vi "test_BuildAdvancedAssets.vi"() -> (3 "Pass?":bool)   [LabVIEW 2019, in "Tests.SolutionBuilder.lvlib"]
uses:
  Tests.SolutionBuilder.lvlib
panel:
  out "test results":u32 format="%03b"
  out "error out":errorcluster
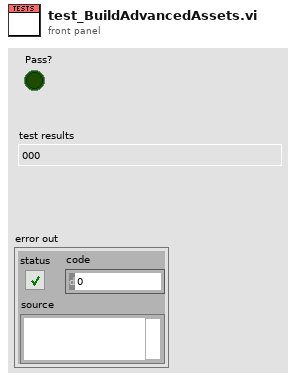
[diagram p1: front panel]
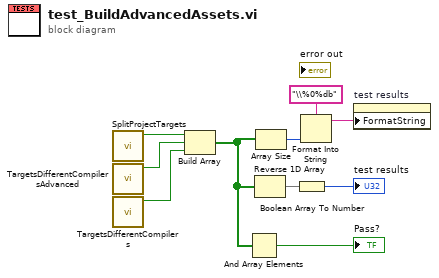
[diagram p0: block diagram]
diagram:
  n1 = call "SplitProjectTargets.vi"() -> ("Pass?"=w6:bool)  [unwired: 11 in]
  n2 = call "TargetsDifferentCompilersAdvanced.vi"() -> ("Pass?"=w1:bool)  [unwired: 10 in, 1 out]
  n3 = call "TargetsDifferentCompilers.vi"() -> ("Pass?"=w5:bool)  [unwired: 11 in]
  n4 = Build Array(w6, w1, w5) -> (w10:bool[])
  n5 = And Array Elements(Boolean array=w10) -> (logical AND=→"Pass?":bool)
  n6 = Reverse 1D Array(array=w10) -> (reversed array=w7:bool[])
  n7 = Array Size(array=w10) -> (size(s)=w8:i32)
  n8 = Boolean Array To Number(Boolean array=w7) -> (number=→"test results":u32)
  n9 = Format Into String(format string="\\%0%db", w8) -> (resulting string=w2:string)  [unwired: 2 in, 1 out]
  n10 = property on="test results" class="DigNum (strict)"("FormatString"=w2) -> ()  [unwired: 2 in, 2 out]
